vi "CC Update Status Values.vi"(8 "error in (no error)":errorcluster, 9 "Values":dbl[](array[numeric]), 10 "names":string[](array[string]), 11 "Data Q":refnum<queue>) -> (0 "error out":errorcluster)   [LabVIEW 2021]
uses:
  Subsystems/SS cluster Data Queue type.ctl
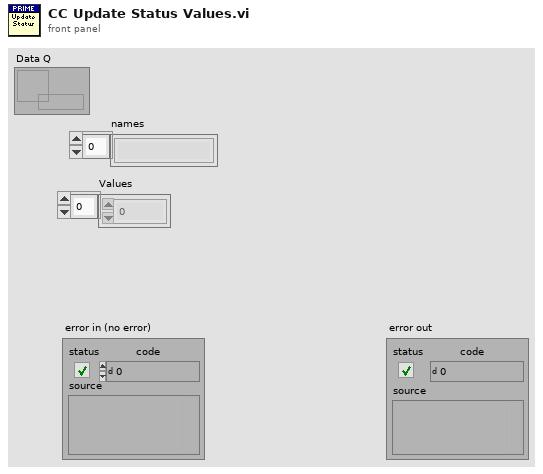
[diagram p1: front panel]
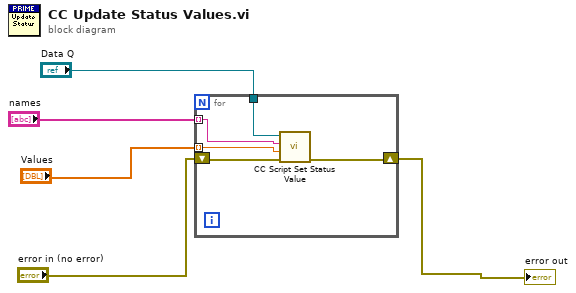
[diagram p0: block diagram]
diagram:
  n1 = for {
    tunnel: "Data Q" -> [w10]
    shift-right: [w8] -> w3
    shift-left: "error in (no error)" -> [w9]
    tunnel: "Values" -> [w7] mode=indexing
    tunnel: "names" -> [w6] mode=indexing
    n2 = call "CC Script Set Status Value.vi"("error in (no error)"=w9, "Value"=w7, "Ch Name"=w6, "Data Q"=w10) -> ("error out"=w8:errorcluster)  [unwired: 7 in]
  }
  "error out" <- w3
